vi "Convert Domain.vi"(8 "Direction":enum16{"Unit", "Real"}(ring), 11 "Real":dbl[](array[numeric])=[0.2787992127517914, 0.23659680929450513, 31.17904685885661]) -> (3 "Unit":dbl[](array[numeric])=[0.27179336078925975, 0.23227872800692473, 0.5177141669170274])   [LabVIEW 2017]
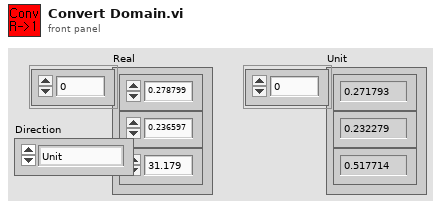
[diagram p1: front panel]
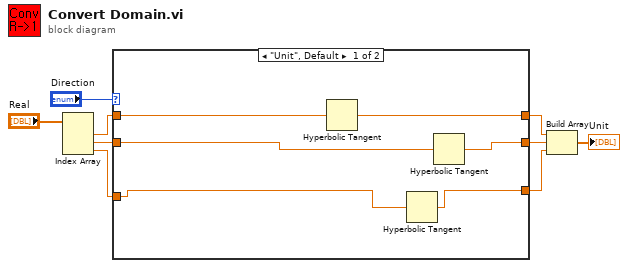
[diagram p0: block diagram]
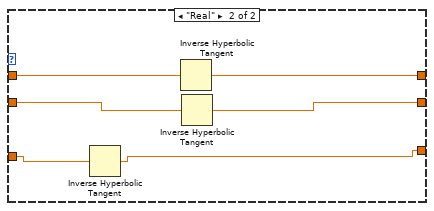
[diagram p2: hidden frame]
diagram:
  n1 = Index Array(array="Real") -> (element #1=w6:dbl, element #2=w7:dbl, element #3=w8:dbl)  [unwired: 3 in]
  n2 = case shown="\"Unit\", Default" "Direction" {
    tunnel: w8 -> [w11 w17]
    tunnel: w7 -> [w15 w19]
    tunnel: w6 -> [w14 w21]
    tunnel: [w10 w16] -> w4
    tunnel: [w13 w18] -> w3
    tunnel: [w12 w20] -> w2
    frame "Unit", Default {
      n3 = Hyperbolic Tangent(1:w14) -> (0:w12:dbl)
      n4 = Hyperbolic Tangent(1:w11) -> (0:w10:dbl)
      n5 = Hyperbolic Tangent(1:w15) -> (0:w13:dbl)
    }
    frame "Real" {
      n6 = Inverse Hyperbolic Tangent(1:w17) -> (0:w16:dbl)
      n7 = Inverse Hyperbolic Tangent(1:w21) -> (0:w20:dbl)
      n8 = Inverse Hyperbolic Tangent(1:w19) -> (0:w18:dbl)
    }
  }
  n9 = Build Array(w2, w3, w4) -> (→"Unit":dbl[])
